vi "Glyph Index.vi"(8 "error in (no error)":errorcluster, 11 "BetterItem in":refnum<class "BetterItem.lvclass">) -> (0 "error out":errorcluster, 2 "Glyph Index":i32, 3 "BetterItem out":refnum<class "BetterItem.lvclass">)   [LabVIEW 2020, in "BetterDragAndDrop.lvlib" / "BetterItem.lvclass"]
uses:
  BetterItem.lvclass
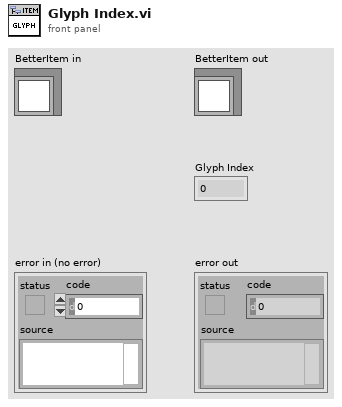
[diagram p1: front panel]
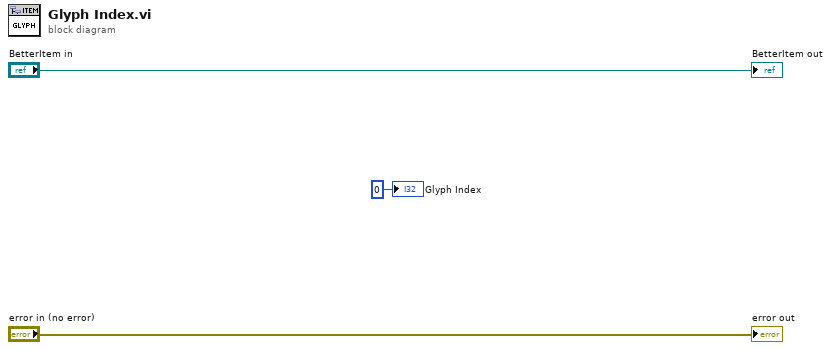
[diagram p0: block diagram]
diagram:
  "error out" <- "error in (no error)"
  "BetterItem out" <- "BetterItem in"
  "Glyph Index" <- 0 ("Glyph Index")
